vi "Error handler.vi"(6 "Test Alarms":u32, 7 "DI no 1 in":u32=6, 8 "Stop Test":bool, 10 "Alarm Input Array":bool[](array[boolean])) -> (0 "Alarm?":bool, 2 "Loop out":u16, 5 "Error no out":dbl=6.0)   [LabVIEW 2014]
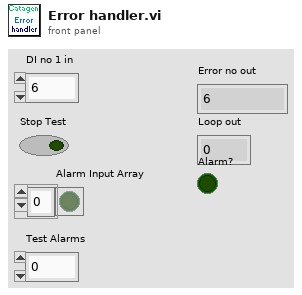
[diagram p1: front panel]
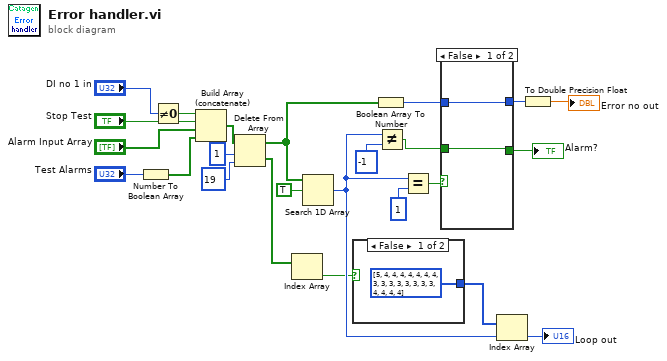
[diagram p0: block diagram]
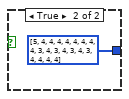
[diagram p2: hidden frame]
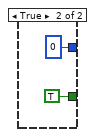
[diagram p3: hidden frame]
diagram:
  n1 = Number To Boolean Array(number="Test Alarms") -> (Boolean array=w7:bool[])
  n2 = Not Equal To 0?(x="DI no 1 in") -> (x != 0?=w11:bool)
  n3 = Build Array (concatenate)(w11, "Stop Test", "Alarm Input Array", w7) -> (w6:bool[])
  n4 = Delete From Array(array=w6, length=1, index=19) -> (deleted portion=w3:bool[], array with subset deleted=w2:bool[])
  n5 = Index Array(array=w3) -> (element=w1:bool)  [unwired: 1 in]
  n6 = Search 1D Array(1D array=w2, element=TRUE) -> (index of element=w17:i32)  [unwired: 1 in]
  n7 = case shown="False" w1 {
    tunnel: [u16[] [5, 4, 4, 4, 4, 4, 4, 4, 3, 3, 3, 3, 3, 3, 3, 3, 4, 4, 4, 4] ("array") u16[] [5, 4, 4, 4, 4, 4, 4, 4, 4, 3, 4, 3, 4, 3, 4, 3, 4, 4, 4, 4] ("array")] -> w10
    frame False {
    }
    frame True {
    }
  }
  n8 = Boolean Array To Number(Boolean array=w2) -> (number=w14:u32)
  n9 = Not Equal?(x=w17, y=-1) -> (x != y?=w20:bool)
  n10 = Equal?(x=w17, y=1) -> (x = y?=w18:bool)
  n11 = case shown="False" w18 {
    tunnel: w20 -> [w28 _]
    tunnel: [w28 TRUE] -> w19
    tunnel: [w27 u32 0] -> w15
    tunnel: w14 -> [w27 _]
    frame False {
    }
    frame True {
    }
  }
  "Alarm?" <- w19
  n12 = Index Array(array=w10, index=w17) -> (element=→"Loop out":u16)
  n13 = To Double Precision Float(number=w15) -> (double precision float=→"Error no out":dbl)
